vi "Toggle.vi"(4 "SetTrue":bool, 6 "SetFalse":bool, 10 "InitialState":bool, 11 "FlashInput":bool) -> (3 "Toggled":bool)   [LabVIEW 2023]
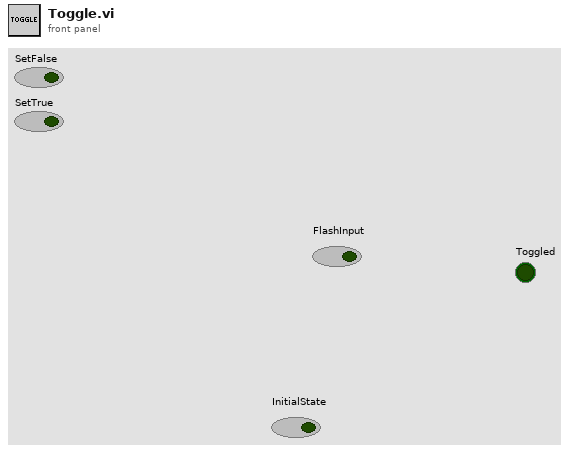
[diagram p1: front panel]
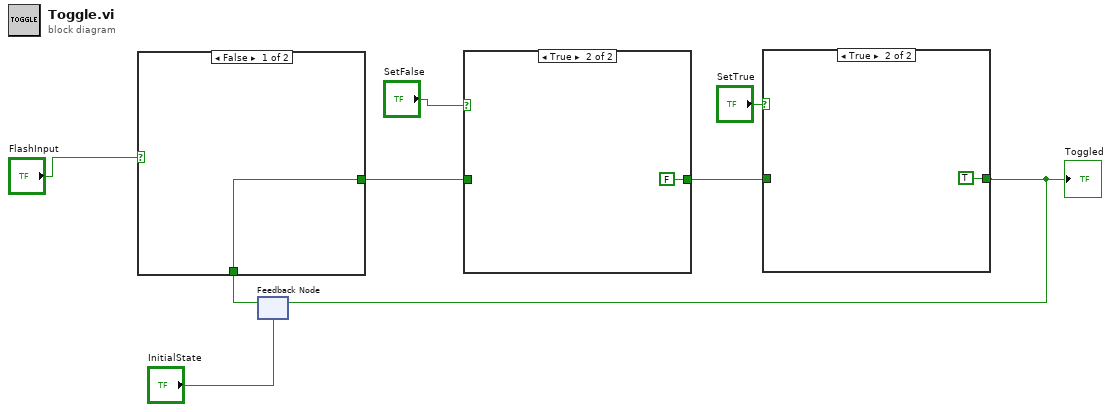
[diagram p0: block diagram]
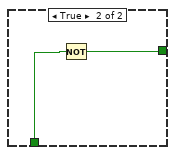
[diagram p4: hidden frame]
diagram:
  n1 = feedback #1("InitialState") -> (w7:bool)
  n2 = case shown="False" "FlashInput" {
    tunnel: [w9 w11] -> w5
    tunnel: w7 -> [w9 w10]
    frame False {
    }
    frame True {
      n3 = Not(x=w10) -> (.not. x?=w11:bool)
    }
  }
  n4 = case shown="True" "SetFalse" {
    tunnel: [w12 FALSE ("InitialState")] -> w3
    tunnel: w5 -> [w12 _]
    frame False {
    }
    frame True {
    }
  }
  n5 = case shown="True" "SetTrue" {
    tunnel: [w14 TRUE ("InitialState")] -> w2
    tunnel: w3 -> [w14 _]
    frame False {
    }
    frame True {
    }
  }
  "Toggled" <- w2
  n6 = feedback-in #1(w2) -> ()
